vi "udp left arm convert.vi"() -> ()   [LabVIEW 2017]
uses:
  global variable.vi
panel:
  out "x-y":i32
  in  "정지":bool
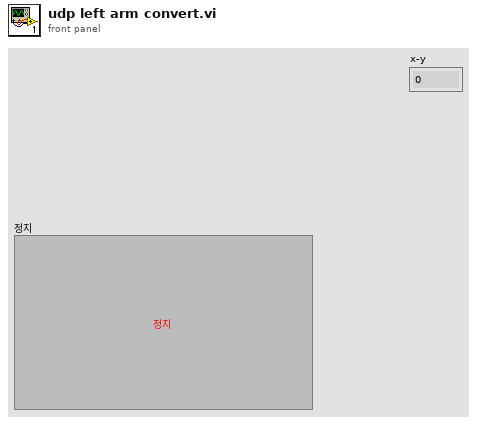
[diagram p1: front panel]
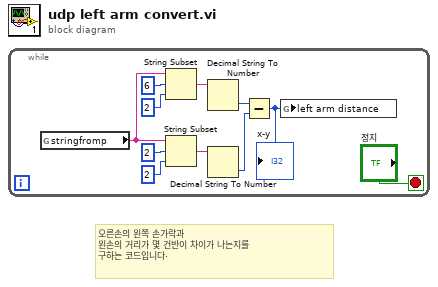
[diagram p0: block diagram]
diagram:
  # "오른손의 왼쪽 손가락과\n왼손의 거리가 몇 건반이 차이가 나는지를\n구하는 코드입니다."
  n1 = while {
    stop <- "정지" stop-if-true
    n2 = global read "global variable.vi" "stringfromp"() -> (w7:string)
    n3 = String Subset(string=w7, offset (0)=6 ("오프셋(0)"), length (rest)=2 ("길이(나머지)")) -> (substring=w4:string)
    n4 = String Subset(string=w7, offset (0)=2 ("오프셋(0)"), length (rest)=2 ("길이(나머지)")) -> (substring=w8:string)
    n5 = Decimal String To Number(string=w4) -> (number=w3:i32)  [unwired: 2 in, 1 out]
    n6 = Decimal String To Number(string=w8) -> (number=w2:i32)  [unwired: 2 in, 1 out]
    n7 = Subtract(x=w3, y=w2) -> (x-y=w1:i32)
    "x-y" <- w1
    n8 = global write "global variable.vi" "left arm distance"(w1) -> ()
  }
